vi "Versioned Load BDX.vi"(1 "path":path) -> (8 "Overall":cluster{"Time (s)":dbl, "Distance (ft)":dbl}, 9 "Trajectory Meta":cluster{"Drive Type":T3, "Path Type":T4}, 15 "Current Limit":dbl, 16 "Points out":cluster{"x":dbl, "y":dbl, "th":dbl}[](array[cluster]), 17 "Fields":T7 {"Overrides"."Angle Override" step=5.0; "Overrides"."Velocity Override" step=5.0; "Overrides"."Angular Override" step=5.0; "Angular Limits"."Jerk (deg/s^3)" min=0.0 step=1.0; "Angular Limits"."Accel (deg/s^2)" min=0.0; "Angular Limits"."Velocity (deg/s)" min=0.0}, 20 "Commands out":T8, 21 "Zero V":bool, 24 "Reversals":T11, 25 "Trajectory Data":T1, 26 "Zero Translational Velocity":bool)   [LabVIEW 2025]
uses:
  Types/Full Command Info.ctl
  Types/Single Cmd Info.ctl
  <vilib>/picture/picture.llb/imagedata.ctl
  Types/Overrides.ctl
  Types/Angluar Limits.ctl
  Types/Drive Type.ctl
  Types/Path Type.ctl
  Types/Trajectory Data.ctl
  Types/Segment Type.ctl
  Types/Availible Command systems for auto.ctl
  Types/Limits.ctl
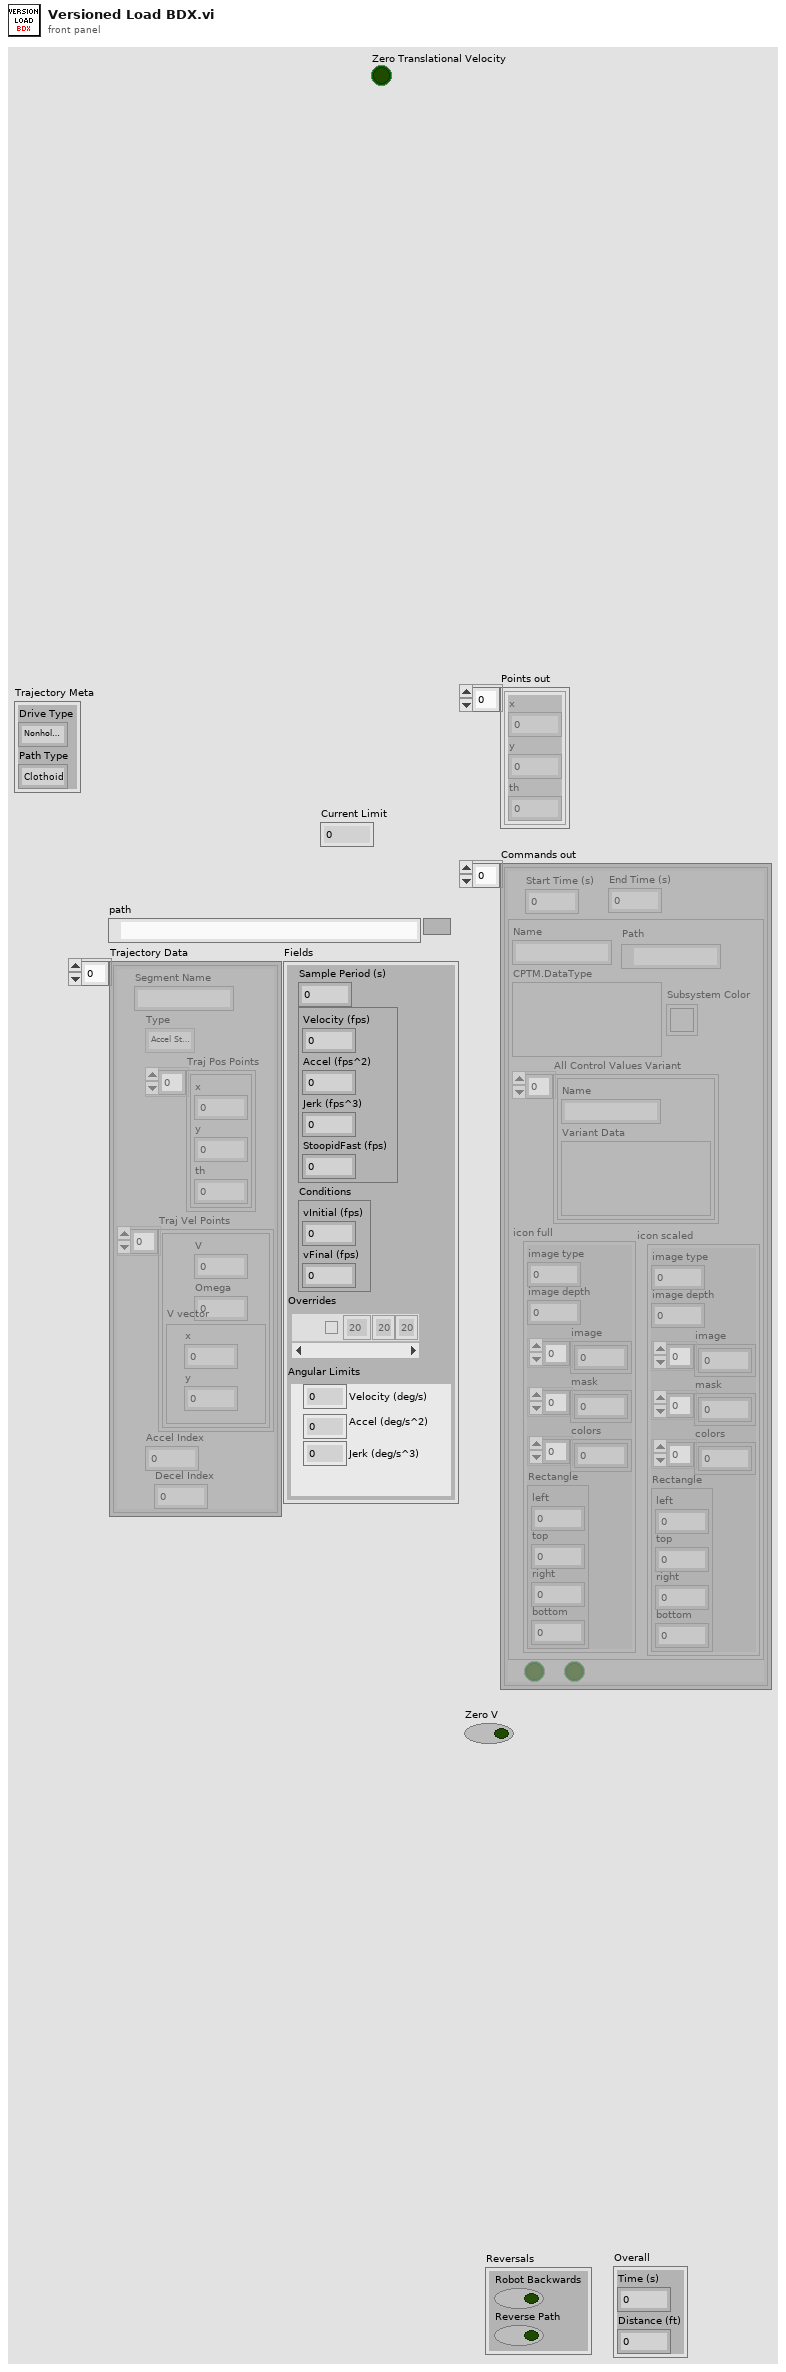
[diagram p1: front panel]
types:
  T1 = typedef "Trajectory Data.ctl" = cluster{"Segment Name":string, "Type":T2, "Traj Pos Points":cluster{"x":dbl, "y":dbl, "th":dbl}[], "Traj Vel Points":cluster{"V":dbl, "Omega":dbl, "V vector":cluster{"y":dbl, "x":dbl}}[], "Accel Index":i32, "Decel Index":i32}[]
  T2 = typedef "Segment Type.ctl" = enum16{"Accel Straight", "Const Straight", "Blend", "Circle", "Bezier"}
  T3 = typedef "Drive Type.ctl" = enum16{"Nonholonomic", "Holonomic"}
  T4 = typedef "Path Type.ctl" = enum16{"Clothoid", "Bezier"}
  T5 = typedef "Overrides.ctl" = cluster{"Count":string, "Angular Override":dbl, "Enabled?":bool, "Velocity Override":dbl, "Angle Override":dbl}[]
  T6 = typedef "Angluar Limits.ctl" = cluster{"Velocity (deg/s)":dbl, "Accel (deg/s^2)":dbl, "Jerk (deg/s^3)":dbl}
  T7 = cluster{"Sample Period (s)":dbl, cluster{"Velocity (fps)":dbl, "Accel (fps^2)":dbl, "Jerk (fps^3)":dbl, "StoopidFast (fps)":dbl}, "Conditions":cluster{"vInitial (fps)":dbl, "vFinal (fps)":dbl}, "Overrides":T5, "Angular Limits":T6}
  T8 = typedef "Full Command Info.ctl" = cluster{"Start Time (s)":dbl, "End Time (s)":dbl, T9, "Visible":bool, "Enabled?":bool}[]
  T9 = typedef "Single Cmd Info.ctl" = cluster{"Name":string, "CPTM.DataType":variant, "All Control Values Variant":cluster{"Name":string, "Variant Data":variant}[], "icon full":T10, "icon scaled":T10, "Path":path, "Subsystem Color":u32}
  T10 = typedef "imagedata.ctl" = cluster{"image type":i32, "image depth":i32, "image":u8[], "mask":u8[], "colors":u32[], "Rectangle":cluster{"left":i16, "top":i16, "right":i16, "bottom":i16}}
  T11 = cluster{"Robot Backwards":bool, "Reverse Path":bool}
  T12 = cluster{"Segment Name":string, "Type":T2, "Traj Pos Points":cluster{"x":dbl, "y":dbl, "th":dbl}[], "Traj Vel Points":cluster{"V":dbl, "Omega":dbl}[], "Accel Index":i32, "Decel Index":i32}[]
  T13 = cluster{"Sample Period (s)":dbl, "Limits 2":cluster{"Velocity (fps)":dbl, "Acceleration (fps^2)":dbl, "Jerk (fps^3)":dbl}, "Conditions":cluster{"vInitial (fps)":dbl, "vFinal (fps)":dbl}, " Acceleration Overrides":cluster{"Angular \nAccelerations":dbl[], "Accel Override Bools":bool[]}}
  T14 = cluster{"Velocity":dbl, "Sample Time":dbl, "Accel":dbl}
  T15 = cluster{"Sample Period (s)":dbl, "Limits":cluster{"Velocity (fps)":dbl, "Acceleration (fps^2)":dbl, "Jerk (fps^3)":dbl}, "Conditions":cluster{"vInitial (fps)":dbl, "vFinal (fps)":dbl}}
  T16 = cluster{"Sample Period (s)":dbl, "Limits":cluster{"Velocity (fps)":dbl, "Acceleration (fps^2)":dbl, "Jerk (fps^3)":dbl}, "Conditions":cluster{"vInitial (fps)":dbl, "vFinal (fps)":dbl}, "Min Rads":dbl[]}
  T17 = typedef "Availible Command systems for auto.ctl" = u16
  T18 = cluster{"Time into Path":dbl, "System":T17, "Item Selected?":bool, "System Selection":T17}[]
  T19 = cluster{"Sample Period (s)":dbl, "Limits 2":cluster{"Velocity (fps)":dbl, "Acceleration (fps^2)":dbl, "Jerk (fps^3)":dbl, "Stoopid Fast":dbl}, "Conditions":cluster{"vInitial (fps)":dbl, "vFinal (fps)":dbl}, " Acceleration Overrides":cluster{"Angular \nAccelerations":dbl[], "Accel Override Bools":bool[]}}
  T20 = cluster{"Sample Period (s)":dbl, "Limits":cluster{"Velocity (fps)":dbl, "Accel (fps^2)":dbl, "Turn Accel (fps^2)":dbl, "Jerk (fps^3)":dbl}, "Conditions":cluster{"vInitial (fps)":dbl, "vFinal (fps)":dbl}, cluster{dbl[], bool[]}}
  T21 = cluster{"Reverse Path":bool, "Robot Backwards":bool}
  T22 = typedef "Limits.ctl" = cluster{"Velocity (fps)":dbl, "Accel (fps^2)":dbl, "Jerk (fps^3)":dbl, "StoopidFast (fps)":dbl}
  T23 = cluster{"Sample Period (s)":dbl, "Limits":T22, "Conditions":cluster{"vInitial (fps)":dbl, "vFinal (fps)":dbl}, "Overrides":T5, "Angular Limits":T6}
  T24 = cluster{"Start Time (s)":dbl, "End Time (s)":dbl, T9, "Visible":bool, "Enabled?":bool}[]
  T25 = cluster{"Velocity":dbl, "Accel":dbl, "Accel":dbl, "Velocity":dbl}
  T26 = cluster{"Velocity (fps)":dbl, "Acceleration (fps^2)":dbl, "Jerk (fps^3)":dbl}
  T27 = cluster{"vInitial (fps)":dbl, "vFinal (fps)":dbl}
  T28 = cluster{"Velocity (fps)":dbl, "Acceleration (fps^2)":dbl, "Jerk (fps^3)":dbl, "Velocity (fps)":dbl}
  T29 = cluster{string, "Angular Multiplier":dbl, bool, "Velocity (fps)":dbl, "Velocity (fps)":dbl}
  T30 = cluster{"Angular \nAccelerations":dbl[], "Accel Override Bools":bool[]}
  T31 = cluster{"Velocity (fps)":dbl, "Acceleration (fps^2)":dbl, "Jerk (fps^3)":dbl, "Stoopid Fast":dbl}
  T32 = cluster{"Velocity (fps)":dbl, "Accel (fps^2)":dbl, "Turn Accel (fps^2)":dbl, "Jerk (fps^3)":dbl}
  T33 = cluster{"Velocity (fps)":dbl, "Accel (fps^2)":dbl, "Jerk (fps^3)":dbl, "StoopidFast (fps)":dbl}
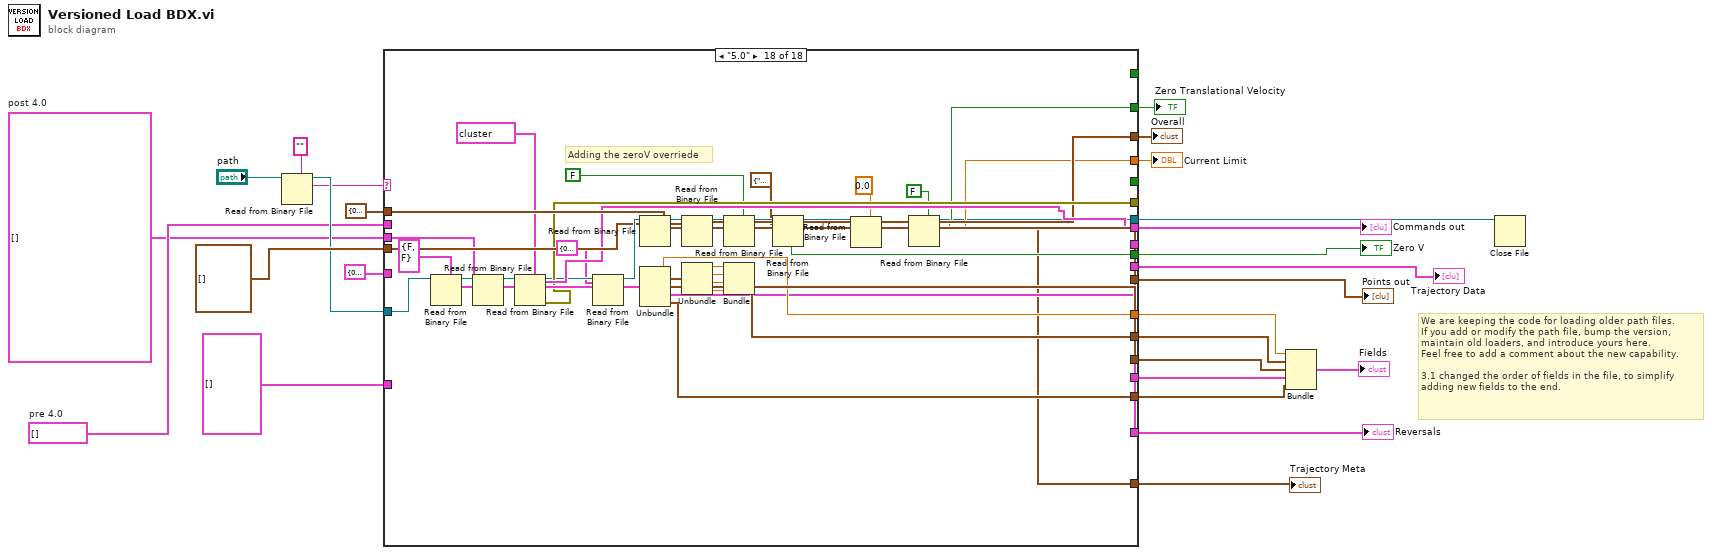
[diagram p0: block diagram]
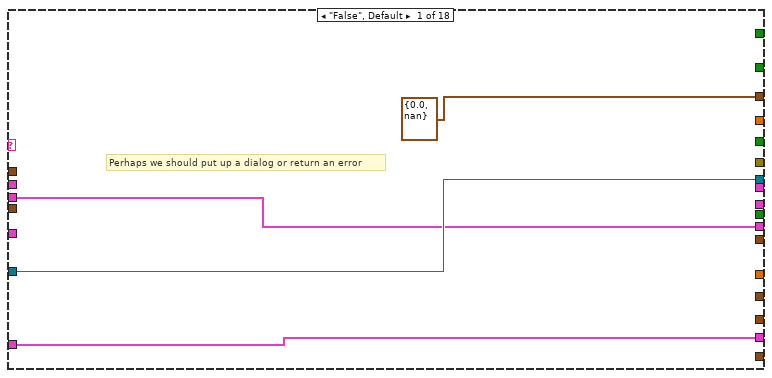
[diagram p2: hidden frame]
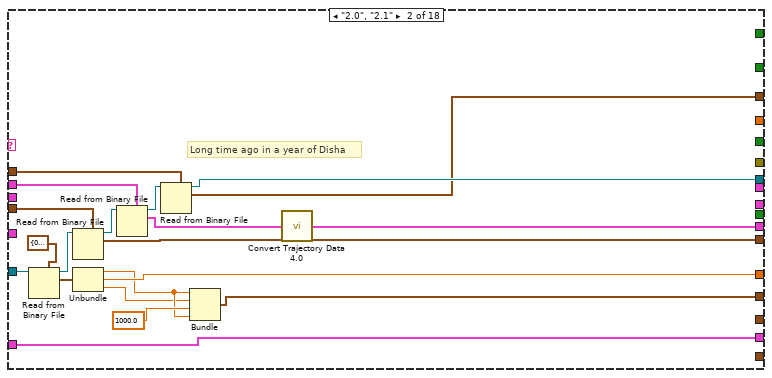
[diagram p3: hidden frame]
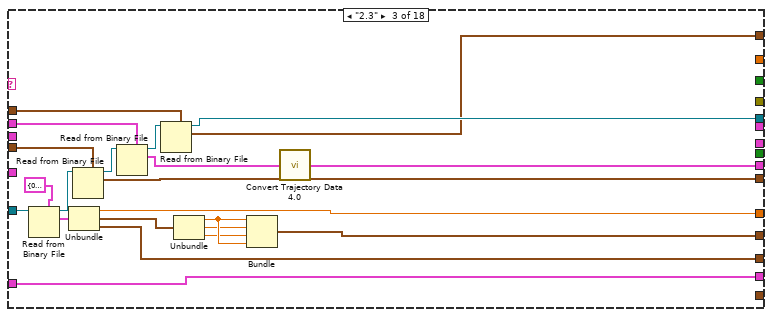
[diagram p4: hidden frame]
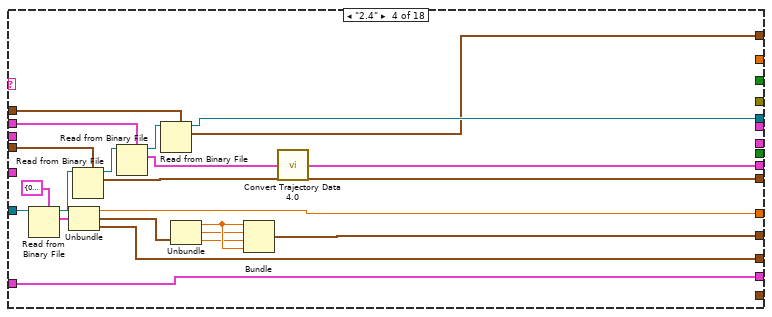
[diagram p5: hidden frame]
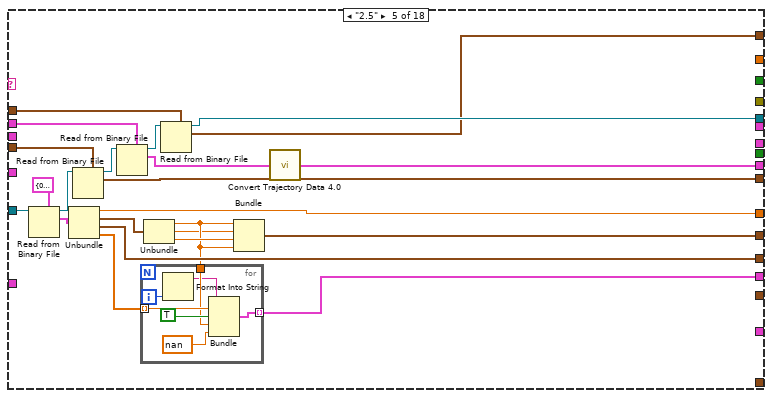
[diagram p6: hidden frame]
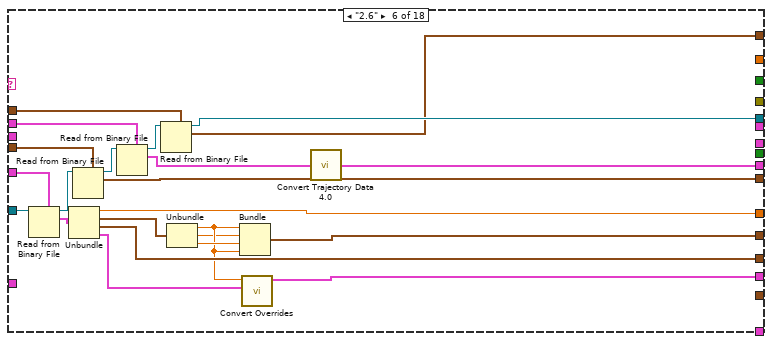
[diagram p7: hidden frame]
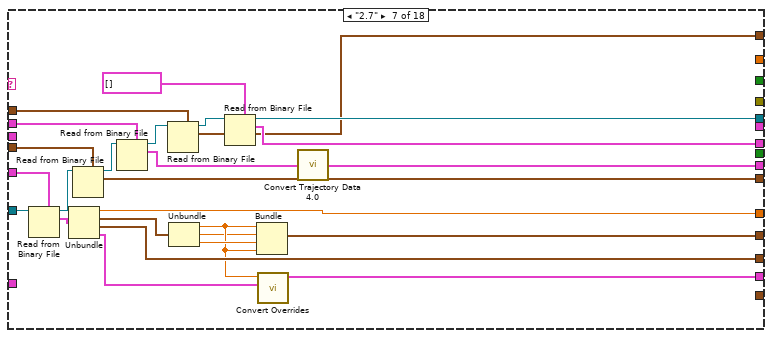
[diagram p8: hidden frame]
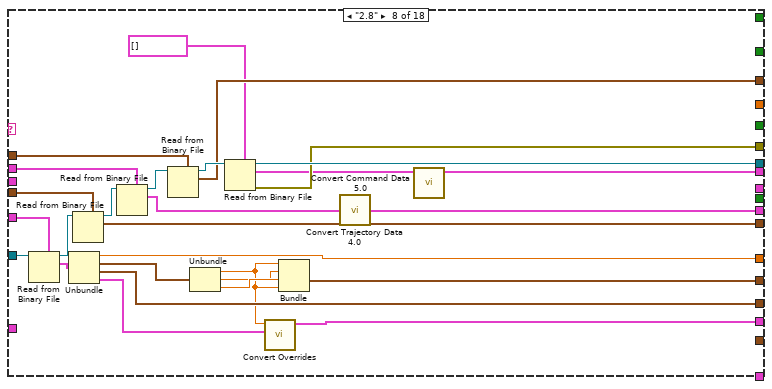
[diagram p9: hidden frame]
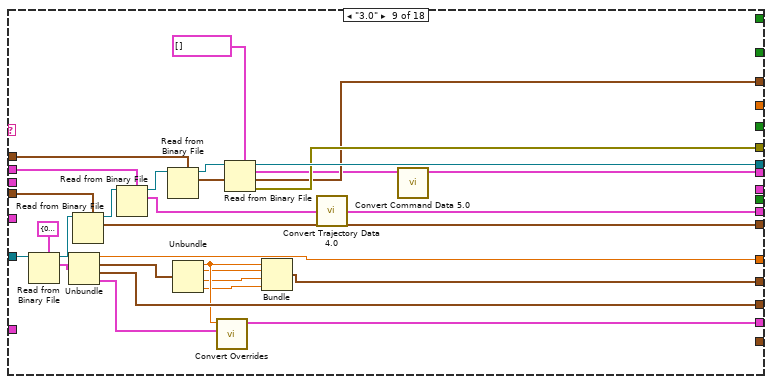
[diagram p10: hidden frame]
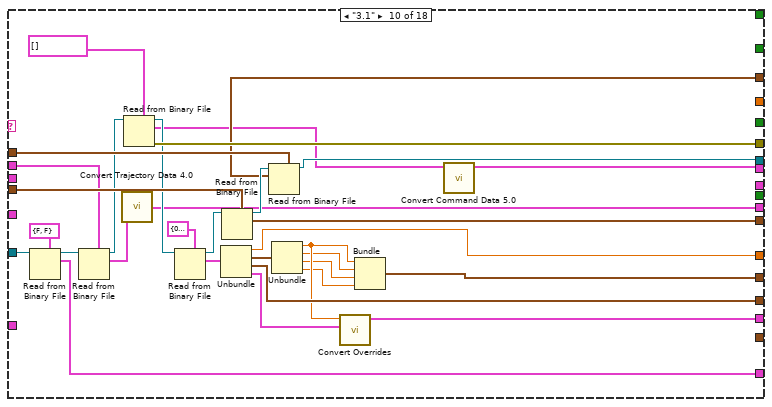
[diagram p11: hidden frame]
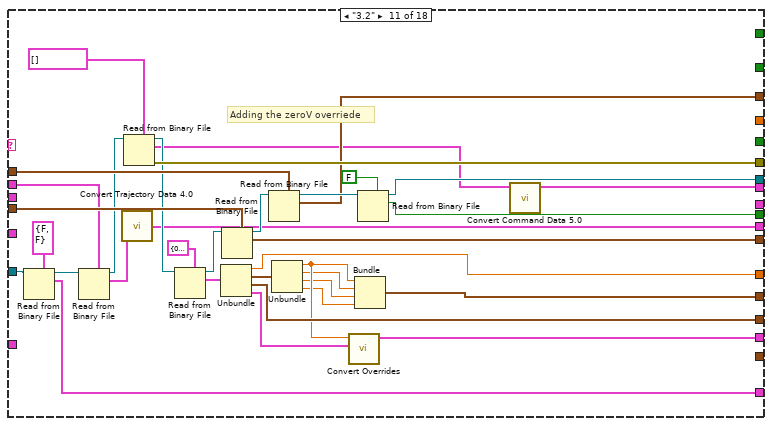
[diagram p12: hidden frame]
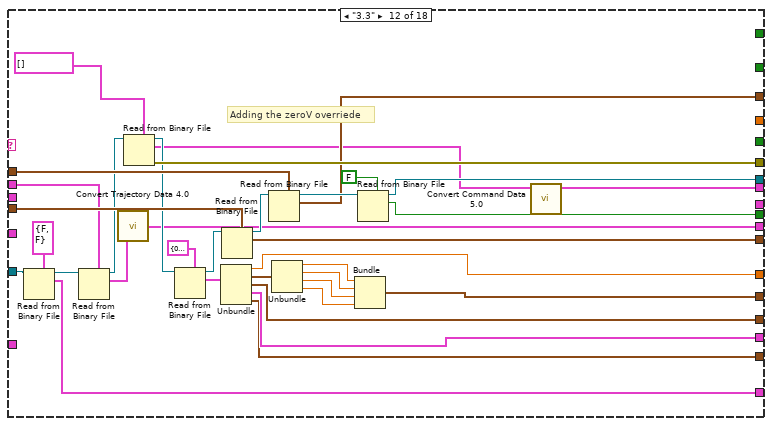
[diagram p13: hidden frame]
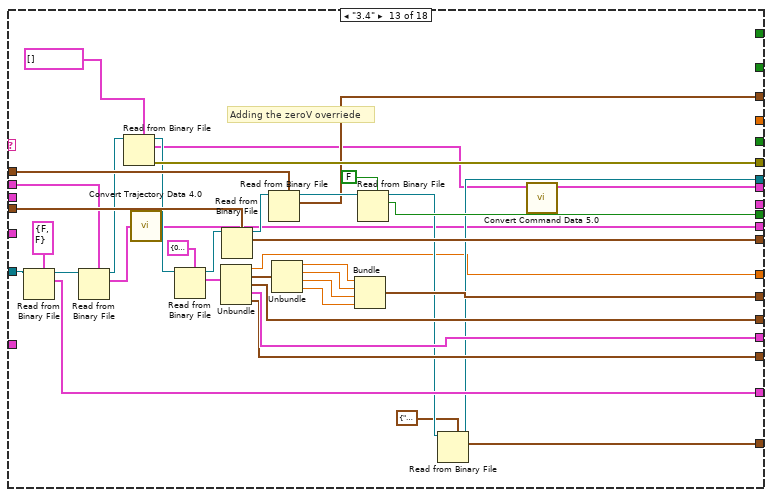
[diagram p14: hidden frame]
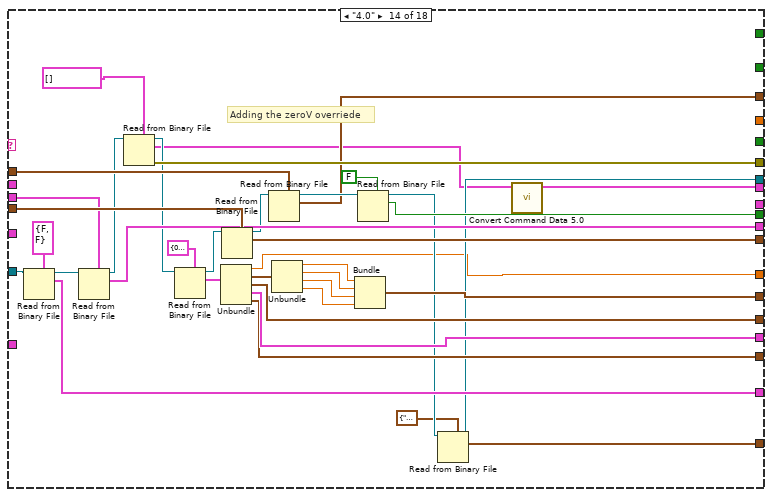
[diagram p15: hidden frame]
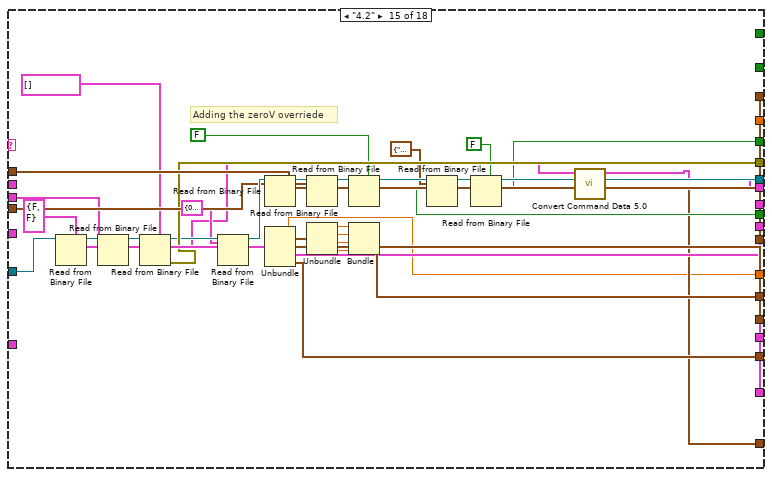
[diagram p16: hidden frame]
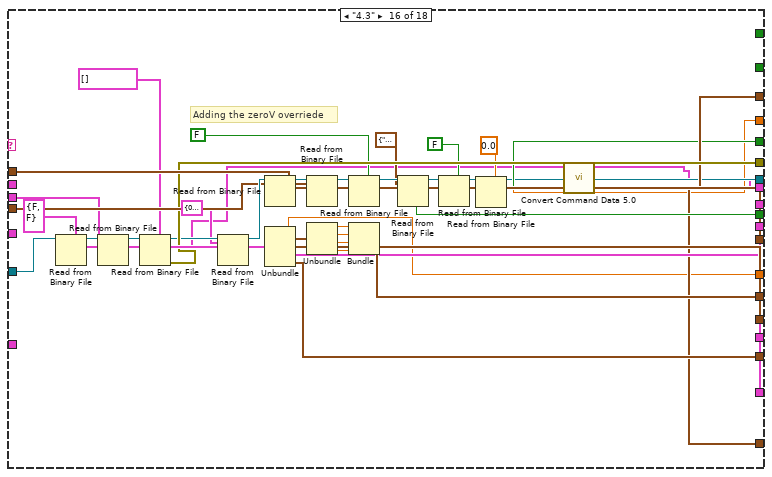
[diagram p17: hidden frame]
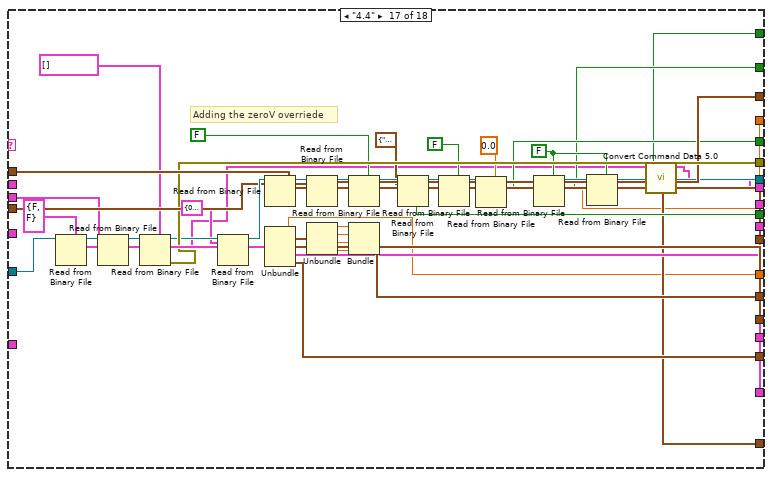
[diagram p18: hidden frame]
diagram:
  w5 = T12 []  # pre 4.0
  w4 = T1 []  # post 4.0
  # "We are keeping the code for loading older path files.\nIf you add or modify the path file, bump the version,\nmaintain old loaders, and introduce yours here.\nFeel free to add a comment about the new capability.\n\n3.1 changed the order of fields in the file, to simplify\nadding new fields to the end."
  n1 = Read from Binary File(5:"" ("String"), 11:"path") -> (2:w11:string, 3:w12:refnum<file>)  [unwired: 4 in, 2 out]
  n2 = case shown="\"5.0\"" w11 {
    tunnel: w12 -> [w30 w49 w71 w93 w116 w146 w172 w200 w229 w253 w288 w323 w361 w399 w439 w482 w530 w571]
    tunnel: cluster{"x":dbl, "y":dbl, "th":dbl}[] [] ("Points in") -> [_ w47 w69 w91 w114 w144 w170 w198 w227 w260 w295 w330 w368 w405 w445 w488 w536 w578]
    tunnel: [_ w46 w68 w90 w113 w143 w169 w197 w226 w259 w294 w329 w367 w404 w444 w487 w535 w577] -> w17
    tunnel: w5 -> [_ w45 w67 w89 w112 w142 w168 w196 w225 w258 w293 w328 w366 _ _ _ _ _]
    tunnel: cluster{"Time (s)":dbl, "Distance (ft)":dbl} {"Time (s)"=0.0, "Distance (ft)"=0.0} ("Cluster 4") -> [_ w43 w65 w87 w110 w140 w166 w194 w223 w257 w292 w327 w365 w403 w443 w486 w534 w576]
    tunnel: [w30 w41 w63 w85 w108 w138 w160 w189 w218 w249 w271 w309 w339 w377 w414 w454 w495 w541] -> w14
    tunnel: [_ w39 w62 w84 w107 w137 w164 w174 w202 w233 w263 w298 w333 w372 w408 w448 w491 w558] -> w23
    tunnel: [_ w35 w56 w77 w101 w132 w154 w186 w208 w241 w277 w315 w353 w391 w431 w474 w522 w563] -> w24
    tunnel: [_ _ w61 w83 w106 w136 w163 w192 w221 w256 w291 w326 w364 w402 w442 w485 w533 w575] -> w25
    tunnel: [w29 w34 w55 w76 w100 w130 w151 w183 w214 w245 w281 w304 w343 w381 w421 w464 w512 w552] -> w26
    tunnel: [w27 w31 w51 w73 w95 w125 w148 w178 w206 w235 w267 w302 w337 w401 w441 w484 w532 w574] -> w3
    tunnel: [_ _ _ _ _ _ w159 _ _ _ _ _ _ _ _ _ _ _] -> _
    tunnel: [_ _ _ _ _ _ _ w175 w203 w231 w264 w299 w334 w371 w409 w449 w493 w573] -> w18
    tunnel: [_ _ _ _ _ _ _ w188 w217 w254 w289 w324 w362 w400 w440 w483 w531 w572] -> _
    tunnel: T13 {"Sample Period (s)"=0.0, "Limits 2"={"Velocity (fps)"=0.0, "Acceleration (fps^2)"=0.0, "Jerk (fps^3)"=0.0}, "Conditions"={"vInitial (fps)"=0.0, "vFinal (fps)"=0.0}, " Acceleration Overrides"={"Angular \nAccelerations"=[], "Accel Override Bools"=[]}} ("Cluster") -> [_ _ _ _ _ w134 w157 w184 _ _ _ _ _ _ _ _ _ _]
    tunnel: [_ _ _ _ _ _ _ _ _ w244 w280 w317 w355 w393 w433 w476 w524 w565] -> w20
    tunnel: T5 [] ("Overrides") -> [w29 w34 w55 w76 _ _ _ _ _ _ _ _ _ _ _ _ _ _]
    tunnel: [_ _ _ _ _ _ _ _ _ _ w269 w307 w346 w384 w424 w467 w515 w555] -> w21
    tunnel: [cluster{"Time (s)":dbl, "Distance (ft)":dbl} {"Time (s)"=0.0, "Distance (ft)"=nan} ("Cluster 4") w32 w52 w74 w96 w126 w149 w179 w207 w236 w268 w306 w345 w383 w423 w466 w514 w554] -> w9
    tunnel: [_ _ _ _ _ _ _ _ _ _ _ w303 w342 w380 w420 w463 w511 w551] -> w7
    tunnel: [_ _ _ _ _ _ _ _ _ _ _ _ w338 w376 w417 w460 w508 w548] -> w6
    tunnel: w4 -> [w27 _ _ _ _ _ _ _ _ _ _ _ _ w375 w416 w459 w507 w547]
    tunnel: [_ _ _ _ _ _ _ _ _ _ _ _ _ _ w412 w456 w504 _] -> _
    tunnel: [_ _ _ _ _ _ _ _ _ _ _ _ _ _ _ w452 w501 w545] -> w2
    tunnel: [_ _ _ _ _ _ _ _ _ _ _ _ _ _ _ _ w497 w542] -> w1
    tunnel: [_ _ _ _ _ _ _ _ _ _ _ _ _ _ _ _ w496 _] -> _
    frame "False", Default {
      # "Perhaps we should put up a dialog or return an error"
    }
    frame "2.0", "2.1" {
      # "Long time ago in a year of Disha"
      n3 = Read from Binary File(5:T14 {"Velocity"=0.0, "Sample Time"=0.0, "Accel"=0.0}, 11:w49) -> (2:w50:T14, 3:w48:refnum<file>)  [unwired: 4 in, 2 out]
      n4 = Read from Binary File(5:w47, 11:w48) -> (2:w46:cluster{"x":dbl, "y":dbl, "th":dbl}[], 3:w44:refnum<file>)  [unwired: 4 in, 2 out]
      n5 = Unbundle(w50) -> ("Velocity"=w36:dbl, "Sample Time"=w39:dbl, "Accel"=w33:dbl)
      n6 = Read from Binary File(5:w45, 11:w44) -> (2:w37:T12, 3:w42:refnum<file>)  [unwired: 4 in, 2 out]
      n7 = Read from Binary File(5:w43, 11:w42) -> (2:w32:cluster{"Time (s)":dbl, "Distance (ft)":dbl}, 3:w41:refnum<file>)  [unwired: 4 in, 2 out]
      n8 = Bundle("Velocity"=w36, "Accel"=w33, "Accel"=1000.0, "Velocity"=w36) -> (w35:T25)  [unwired: 1 in]
      n9 = call "Convert Trajectory Data 4.0.vi"("pre 4.0"=w37) -> ("post 4.0"=w31:T1)
    }
    frame "2.3" {
      n10 = Read from Binary File(5:T15 {"Sample Period (s)"=0.0, "Limits"={"Velocity (fps)"=0.0, "Acceleration (fps^2)"=0.0, "Jerk (fps^3)"=0.0}, "Conditions"={"vInitial (fps)"=0.0, "vFinal (fps)"=0.0}}, 11:w71) -> (2:w72:T15, 3:w70:refnum<file>)  [unwired: 4 in, 2 out]
      n11 = Unbundle(w72) -> ("Sample Period (s)"=w62:dbl, "Limits"=w53:T26, "Conditions"=w61:T27)
      n12 = Read from Binary File(5:w69, 11:w70) -> (2:w68:cluster{"x":dbl, "y":dbl, "th":dbl}[], 3:w66:refnum<file>)  [unwired: 4 in, 2 out]
      n13 = Read from Binary File(5:w67, 11:w66) -> (2:w59:T12, 3:w64:refnum<file>)  [unwired: 4 in, 2 out]
      n14 = Read from Binary File(5:w65, 11:w64) -> (2:w52:cluster{"Time (s)":dbl, "Distance (ft)":dbl}, 3:w63:refnum<file>)  [unwired: 4 in, 2 out]
      n15 = Unbundle(w53) -> ("Velocity (fps)"=w58:dbl, "Acceleration (fps^2)"=w54:dbl, "Jerk (fps^3)"=w57:dbl)
      n16 = Bundle("Velocity (fps)"=w58, "Acceleration (fps^2)"=w54, "Jerk (fps^3)"=w57, "Velocity (fps)"=w58) -> (w56:T28)  [unwired: 1 in]
      n17 = call "Convert Trajectory Data 4.0.vi"("pre 4.0"=w59) -> ("post 4.0"=w51:T1)
    }
    frame "2.4" {
      n18 = Read from Binary File(5:T15 {"Sample Period (s)"=0.0, "Limits"={"Velocity (fps)"=0.0, "Acceleration (fps^2)"=0.0, "Jerk (fps^3)"=0.0}, "Conditions"={"vInitial (fps)"=0.0, "vFinal (fps)"=0.0}}, 11:w93) -> (2:w94:T15, 3:w92:refnum<file>)  [unwired: 4 in, 2 out]
      n19 = Unbundle(w94) -> ("Sample Period (s)"=w84:dbl, "Limits"=w78:T26, "Conditions"=w83:T27)
      n20 = Read from Binary File(5:w91, 11:w92) -> (2:w90:cluster{"x":dbl, "y":dbl, "th":dbl}[], 3:w88:refnum<file>)  [unwired: 4 in, 2 out]
      n21 = Read from Binary File(5:w89, 11:w88) -> (2:w81:T12, 3:w86:refnum<file>)  [unwired: 4 in, 2 out]
      n22 = Read from Binary File(5:w87, 11:w86) -> (2:w74:cluster{"Time (s)":dbl, "Distance (ft)":dbl}, 3:w85:refnum<file>)  [unwired: 4 in, 2 out]
      n23 = Unbundle(w78) -> ("Velocity (fps)"=w80:dbl, "Acceleration (fps^2)"=w75:dbl, "Jerk (fps^3)"=w79:dbl)
      n24 = Bundle("Velocity (fps)"=w80, "Acceleration (fps^2)"=w75, "Jerk (fps^3)"=w79, "Velocity (fps)"=w80) -> (w77:T28)  [unwired: 1 in]
      n25 = call "Convert Trajectory Data 4.0.vi"("pre 4.0"=w81) -> ("post 4.0"=w73:T1)
    }
    frame "2.5" {
      n26 = Read from Binary File(5:T16 {"Sample Period (s)"=0.0, "Limits"={"Velocity (fps)"=0.0, "Acceleration (fps^2)"=0.0, "Jerk (fps^3)"=0.0}, "Conditions"={"vInitial (fps)"=0.0, "vFinal (fps)"=0.0}, "Min Rads"=[20.0, 20.0, 20.0, 20.0, 20.0]}, 11:w116) -> (2:w117:T16, 3:w115:refnum<file>)  [unwired: 4 in, 2 out]
      n27 = Unbundle(w117) -> ("Sample Period (s)"=w107:dbl, "Limits"=w102:T26, "Conditions"=w106:T27, "Min Rads"=w99:dbl[])
      n28 = Read from Binary File(5:w114, 11:w115) -> (2:w113:cluster{"x":dbl, "y":dbl, "th":dbl}[], 3:w111:refnum<file>)  [unwired: 4 in, 2 out]
      n29 = Read from Binary File(5:w112, 11:w111) -> (2:w104:T12, 3:w109:refnum<file>)  [unwired: 4 in, 2 out]
      n30 = Unbundle(w102) -> ("Velocity (fps)"=w98:dbl, "Acceleration (fps^2)"=w97:dbl, "Jerk (fps^3)"=w103:dbl)
      n31 = for {
        tunnel: [w123] -> w100 mode=indexing
        tunnel: w99 -> [w122] mode=indexing
        tunnel: w98 -> [w121]
        i -> [w120]
        n32 = Format Into String(w120) -> (resulting string=w119:string)  [unwired: 3 in, 1 out]
        n33 = Bundle(w119, "Angular Multiplier"=w122, TRUE, "Velocity (fps)"=w121, "Velocity (fps)"=nan) -> (w123:T29)  [unwired: 1 in]
      }
      n34 = Read from Binary File(5:w110, 11:w109) -> (2:w96:cluster{"Time (s)":dbl, "Distance (ft)":dbl}, 3:w108:refnum<file>)  [unwired: 4 in, 2 out]
      n35 = Bundle("Velocity (fps)"=w98, "Acceleration (fps^2)"=w97, "Jerk (fps^3)"=w103, "Velocity (fps)"=w98) -> (w101:T28)  [unwired: 1 in]
      n36 = call "Convert Trajectory Data 4.0.vi"("pre 4.0"=w104) -> ("post 4.0"=w95:T1)
    }
    frame "2.6" {
      n37 = Read from Binary File(5:w134, 11:w146) -> (2:w147:T13, 3:w145:refnum<file>)  [unwired: 4 in, 2 out]
      n38 = Unbundle(w147) -> ("Sample Period (s)"=w137:dbl, "Limits 2"=w131:T26, "Conditions"=w136:T27, "Acceleration Overrides"=w128:T30)
      n39 = Read from Binary File(5:w144, 11:w145) -> (2:w143:cluster{"x":dbl, "y":dbl, "th":dbl}[], 3:w141:refnum<file>)  [unwired: 4 in, 2 out]
      n40 = Read from Binary File(5:w142, 11:w141) -> (2:w135:T12, 3:w139:refnum<file>)  [unwired: 4 in, 2 out]
      n41 = Read from Binary File(5:w140, 11:w139) -> (2:w126:cluster{"Time (s)":dbl, "Distance (ft)":dbl}, 3:w138:refnum<file>)  [unwired: 4 in, 2 out]
      n42 = Unbundle(w131) -> ("Velocity (fps)"=w129:dbl, "Acceleration (fps^2)"=w127:dbl, "Jerk (fps^3)"=w133:dbl)
      n43 = Bundle("Velocity (fps)"=w129, "Acceleration (fps^2)"=w127, "Jerk (fps^3)"=w133, "Velocity (fps)"=w129) -> (w132:T28)  [unwired: 1 in]
      n44 = call "Convert Overrides.vi"("Cluster"=w128, "Velocity (fps)"=w129) -> ("Overrides"=w130:T5)  [unwired: 9 in]
      n45 = call "Convert Trajectory Data 4.0.vi"("pre 4.0"=w135) -> ("post 4.0"=w125:T1)
    }
    frame "2.7" {
      n46 = Read from Binary File(5:w157, 11:w172) -> (2:w173:T13, 3:w171:refnum<file>)  [unwired: 4 in, 2 out]
      n47 = Unbundle(w173) -> ("Sample Period (s)"=w164:dbl, "Limits 2"=w155:T26, "Conditions"=w163:T27, "Acceleration Overrides"=w152:T30)
      n48 = Read from Binary File(5:w170, 11:w171) -> (2:w169:cluster{"x":dbl, "y":dbl, "th":dbl}[], 3:w167:refnum<file>)  [unwired: 4 in, 2 out]
      n49 = Read from Binary File(5:w168, 11:w167) -> (2:w162:T12, 3:w165:refnum<file>)  [unwired: 4 in, 2 out]
      n50 = Read from Binary File(5:w166, 11:w165) -> (2:w149:cluster{"Time (s)":dbl, "Distance (ft)":dbl}, 3:w161:refnum<file>)  [unwired: 4 in, 2 out]
      n51 = Unbundle(w155) -> ("Velocity (fps)"=w153:dbl, "Acceleration (fps^2)"=w150:dbl, "Jerk (fps^3)"=w156:dbl)
      n52 = Read from Binary File(5:T18 [] ("Commands"), 11:w161) -> (2:w159:T18, 3:w160:refnum<file>)  [unwired: 4 in, 2 out]
      n53 = Bundle("Velocity (fps)"=w153, "Acceleration (fps^2)"=w150, "Jerk (fps^3)"=w156, "Velocity (fps)"=w153) -> (w154:T28)  [unwired: 1 in]
      n54 = call "Convert Overrides.vi"("Cluster"=w152, "Velocity (fps)"=w153) -> ("Overrides"=w151:T5)  [unwired: 9 in]
      n55 = call "Convert Trajectory Data 4.0.vi"("pre 4.0"=w162) -> ("post 4.0"=w148:T1)
    }
    frame "2.8" {
      n56 = Read from Binary File(5:w184, 11:w200) -> (2:w201:T13, 3:w199:refnum<file>)  [unwired: 4 in, 2 out]
      n57 = Unbundle(w201) -> ("Sample Period (s)"=w174:dbl, "Limits 2"=w187:T26, "Conditions"=w192:T27, "Acceleration Overrides"=w181:T30)
      n58 = Read from Binary File(5:w198, 11:w199) -> (2:w197:cluster{"x":dbl, "y":dbl, "th":dbl}[], 3:w195:refnum<file>)  [unwired: 4 in, 2 out]
      n59 = Read from Binary File(5:w196, 11:w195) -> (2:w191:T12, 3:w193:refnum<file>)  [unwired: 4 in, 2 out]
      n60 = Read from Binary File(5:w194, 11:w193) -> (2:w179:cluster{"Time (s)":dbl, "Distance (ft)":dbl}, 3:w190:refnum<file>)  [unwired: 4 in, 2 out]
      n61 = Unbundle(w187) -> ("Velocity (fps)"=w182:dbl, "Acceleration (fps^2)"=w180:dbl, "Jerk (fps^3)"=w185:dbl)
      n62 = Read from Binary File(5:cluster{"Time (s)":dbl, T9, bool}[] [] ("Commands in"), 11:w190) -> (0:w188:errorcluster, 2:w176:cluster{"Time (s)":dbl, T9, bool}[], 3:w189:refnum<file>)  [unwired: 4 in, 1 out]
      n63 = call "Convert Overrides.vi"("Cluster"=w181, "Velocity (fps)"=w182) -> ("Overrides"=w183:T5)  [unwired: 9 in]
      n64 = Bundle("Velocity (fps)"=w182, "Acceleration (fps^2)"=w180, "Jerk (fps^3)"=w185, "Velocity (fps)"=w182) -> (w186:T28)  [unwired: 1 in]
      n65 = call "Convert Trajectory Data 4.0.vi"("pre 4.0"=w191) -> ("post 4.0"=w178:T1)
      n66 = call "Convert Command Data 5.0.vi"("Pre 5.0 Command Data"=w176) -> ("5.0 Command Data"=w175:T8)  [unwired: 10 in]
    }
    frame "3.0" {
      n67 = Read from Binary File(5:T19 {"Sample Period (s)"=0.0, "Limits 2"={"Velocity (fps)"=0.0, "Acceleration (fps^2)"=0.0, "Jerk (fps^3)"=0.0, "Stoopid Fast"=0.0}, "Conditions"={"vInitial (fps)"=0.0, "vFinal (fps)"=0.0}, " Acceleration Overrides"={"Angular \nAccelerations"=[], "Accel Override Bools"=[]}} ("Cluster"), 11:w229) -> (2:w230:T19, 3:w228:refnum<file>)  [unwired: 4 in, 2 out]
      n68 = Unbundle(w230) -> ("Sample Period (s)"=w202:dbl, "Limits 2"=w209:T31, "Conditions"=w221:T27, "Acceleration Overrides"=w215:T30)
      n69 = Read from Binary File(5:w227, 11:w228) -> (2:w226:cluster{"x":dbl, "y":dbl, "th":dbl}[], 3:w224:refnum<file>)  [unwired: 4 in, 2 out]
      n70 = Read from Binary File(5:w225, 11:w224) -> (2:w220:T12, 3:w222:refnum<file>)  [unwired: 4 in, 2 out]
      n71 = Read from Binary File(5:w223, 11:w222) -> (2:w207:cluster{"Time (s)":dbl, "Distance (ft)":dbl}, 3:w219:refnum<file>)  [unwired: 4 in, 2 out]
      n72 = Unbundle(w209) -> ("Velocity (fps)"=w213:dbl, "Acceleration (fps^2)"=w212:dbl, "Jerk (fps^3)"=w211:dbl, "Stoopid Fast"=w210:dbl)
      n73 = call "Convert Overrides.vi"("Cluster"=w215, "Velocity (fps)"=w213) -> ("Overrides"=w214:T5)  [unwired: 9 in]
      n74 = Read from Binary File(5:cluster{"Time (s)":dbl, T9, bool}[] [] ("Commands in"), 11:w219) -> (0:w217:errorcluster, 2:w204:cluster{"Time (s)":dbl, T9, bool}[], 3:w218:refnum<file>)  [unwired: 4 in, 1 out]
      n75 = Bundle("Velocity (fps)"=w213, "Acceleration (fps^2)"=w212, "Jerk (fps^3)"=w211, "Stoopid Fast"=w210) -> (w208:T31)  [unwired: 1 in]
      n76 = call "Convert Trajectory Data 4.0.vi"("pre 4.0"=w220) -> ("post 4.0"=w206:T1)
      n77 = call "Convert Command Data 5.0.vi"("Pre 5.0 Command Data"=w204) -> ("5.0 Command Data"=w203:T8)  [unwired: 10 in]
    }
    frame "3.1" {
      n78 = Read from Binary File(5:T21 {"Reverse Path"=FALSE, "Robot Backwards"=FALSE} ("Cluster"), 11:w253) -> (2:w244:T21, 3:w250:refnum<file>)  [unwired: 4 in, 2 out]
      n79 = Read from Binary File(5:w258, 11:w250) -> (2:w255:T12, 3:w248:refnum<file>)  [unwired: 4 in, 2 out]
      n80 = call "Convert Trajectory Data 4.0.vi"("pre 4.0"=w255) -> ("post 4.0"=w235:T1)
      n81 = Read from Binary File(5:cluster{"Time (s)":dbl, T9, bool}[] [] ("Commands in"), 11:w248) -> (0:w254:errorcluster, 2:w232:cluster{"Time (s)":dbl, T9, bool}[], 3:w247:refnum<file>)  [unwired: 4 in, 1 out]
      n82 = Read from Binary File(5:T20 {"Sample Period (s)"=0.0, "Limits"={"Velocity (fps)"=0.0, "Accel (fps^2)"=0.0, "Turn Accel (fps^2)"=15.0, "Jerk (fps^3)"=0.0}, "Conditions"={"vInitial (fps)"=0.0, "vFinal (fps)"=0.0}, {[], []}} ("Cluster 2"), 11:w247) -> (2:w262:T20, 3:w261:refnum<file>)  [unwired: 4 in, 2 out]
      n83 = Unbundle(w262) -> ("Sample Period (s)"=w233:dbl, "Limits"=w243:T32, "Conditions"=w256:T27, w246:cluster{dbl[], bool[]})
      n84 = Read from Binary File(5:w260, 11:w261) -> (2:w259:cluster{"x":dbl, "y":dbl, "th":dbl}[], 3:w251:refnum<file>)  [unwired: 4 in, 2 out]
      n85 = Read from Binary File(5:w257, 11:w251) -> (2:w236:cluster{"Time (s)":dbl, "Distance (ft)":dbl}, 3:w249:refnum<file>)  [unwired: 4 in, 2 out]
      n86 = Unbundle(w243) -> ("Velocity (fps)"=w240:dbl, "Accel (fps^2)"=w239:dbl, "Turn Accel (fps^2)"=w238:dbl, "Jerk (fps^3)"=w237:dbl)
      n87 = call "Convert Overrides.vi"("Cluster"=w246, "Velocity (fps)"=w240) -> ("Overrides"=w245:T5)  [unwired: 9 in]
      n88 = Bundle("Velocity (fps)"=w240, "Accel (fps^2)"=w239, "Turn Accel (fps^2)"=w238, "Jerk (fps^3)"=w237) -> (w241:T32)  [unwired: 1 in]
      n89 = call "Convert Command Data 5.0.vi"("Pre 5.0 Command Data"=w232) -> ("5.0 Command Data"=w231:T8)  [unwired: 10 in]
    }
    frame "3.2" {
      # "Adding the zeroV overriede"
      n90 = Read from Binary File(5:T11 {"Robot Backwards"=FALSE, "Reverse Path"=FALSE} ("Cluster"), 11:w288) -> (2:w280:T11, 3:w285:refnum<file>)  [unwired: 4 in, 2 out]
      n91 = Read from Binary File(5:w293, 11:w285) -> (2:w290:T12, 3:w284:refnum<file>)  [unwired: 4 in, 2 out]
      n92 = call "Convert Trajectory Data 4.0.vi"("pre 4.0"=w290) -> ("post 4.0"=w267:T1)
      n93 = Read from Binary File(5:cluster{"Time (s)":dbl, T9, bool}[] [] ("Commands in"), 11:w284) -> (0:w289:errorcluster, 2:w265:cluster{"Time (s)":dbl, T9, bool}[], 3:w283:refnum<file>)  [unwired: 4 in, 1 out]
      n94 = Read from Binary File(5:T20 {"Sample Period (s)"=0.0, "Limits"={"Velocity (fps)"=0.0, "Accel (fps^2)"=0.0, "Turn Accel (fps^2)"=15.0, "Jerk (fps^3)"=0.0}, "Conditions"={"vInitial (fps)"=0.0, "vFinal (fps)"=0.0}, {[], []}} ("Cluster 2"), 11:w283) -> (2:w297:T20, 3:w296:refnum<file>)  [unwired: 4 in, 2 out]
      n95 = Unbundle(w297) -> ("Sample Period (s)"=w263:dbl, "Limits"=w279:T32, "Conditions"=w291:T27, w282:cluster{dbl[], bool[]})
      n96 = Read from Binary File(5:w295, 11:w296) -> (2:w294:cluster{"x":dbl, "y":dbl, "th":dbl}[], 3:w286:refnum<file>)  [unwired: 4 in, 2 out]
      n97 = Read from Binary File(5:w292, 11:w286) -> (2:w268:cluster{"Time (s)":dbl, "Distance (ft)":dbl}, 3:w272:refnum<file>)  [unwired: 4 in, 2 out]
      n98 = Unbundle(w279) -> ("Velocity (fps)"=w276:dbl, "Accel (fps^2)"=w275:dbl, "Turn Accel (fps^2)"=w274:dbl, "Jerk (fps^3)"=w273:dbl)
      n99 = call "Convert Overrides.vi"("Cluster"=w282, "Velocity (fps)"=w276) -> ("Overrides"=w281:T5)  [unwired: 9 in]
      n100 = Bundle("Velocity (fps)"=w276, "Accel (fps^2)"=w275, "Turn Accel (fps^2)"=w274, "Jerk (fps^3)"=w273) -> (w277:T32)  [unwired: 1 in]
      n101 = Read from Binary File(5:FALSE, 11:w272) -> (2:w269:bool, 3:w271:refnum<file>)  [unwired: 4 in, 2 out]
      n102 = call "Convert Command Data 5.0.vi"("Pre 5.0 Command Data"=w265) -> ("5.0 Command Data"=w264:T8)  [unwired: 10 in]
    }
    frame "3.3" {
      # "Adding the zeroV overriede"
      n103 = Read from Binary File(5:T11 {"Robot Backwards"=FALSE, "Reverse Path"=FALSE} ("Cluster"), 11:w323) -> (2:w317:T11, 3:w320:refnum<file>)  [unwired: 4 in, 2 out]
      n104 = Read from Binary File(5:w328, 11:w320) -> (2:w325:T12, 3:w319:refnum<file>)  [unwired: 4 in, 2 out]
      n105 = call "Convert Trajectory Data 4.0.vi"("pre 4.0"=w325) -> ("post 4.0"=w302:T1)
      n106 = Read from Binary File(5:cluster{"Time (s)":dbl, T9, bool}[] [] ("Commands in"), 11:w319) -> (0:w324:errorcluster, 2:w300:cluster{"Time (s)":dbl, T9, bool}[], 3:w318:refnum<file>)  [unwired: 4 in, 1 out]
      n107 = Read from Binary File(5:T23 {"Sample Period (s)"=0.0, "Limits"={"Velocity (fps)"=0.0, "Accel (fps^2)"=0.0, "Jerk (fps^3)"=0.0, "StoopidFast (fps)"=0.0}, "Conditions"={"vInitial (fps)"=0.0, "vFinal (fps)"=0.0}, "Overrides"=[], "Angular Limits"={"Velocity (deg/s)"=0.0, "Accel (deg/s^2)"=0.0, "Jerk (deg/s^3)"=0.0}} ("output cluster"), 11:w318) -> (2:w332:T23, 3:w331:refnum<file>)  [unwired: 4 in, 2 out]
      n108 = Unbundle(w332) -> ("Sample Period (s)"=w298:dbl, "Limits"=w316:T22, "Conditions"=w326:T27, "Overrides"=w304:T5, "Angular Limits"=w303:T6)
      n109 = Read from Binary File(5:w330, 11:w331) -> (2:w329:cluster{"x":dbl, "y":dbl, "th":dbl}[], 3:w321:refnum<file>)  [unwired: 4 in, 2 out]
      n110 = Read from Binary File(5:w327, 11:w321) -> (2:w306:cluster{"Time (s)":dbl, "Distance (ft)":dbl}, 3:w310:refnum<file>)  [unwired: 4 in, 2 out]
      n111 = Unbundle(w316) -> ("Velocity (fps)"=w314:dbl, "Accel (fps^2)"=w313:dbl, "Jerk (fps^3)"=w312:dbl, "StoopidFast (fps)"=w311:dbl)
      n112 = Bundle("Velocity (fps)"=w314, "Accel (fps^2)"=w313, "Jerk (fps^3)"=w312, "StoopidFast (fps)"=w311) -> (w315:T33)  [unwired: 1 in]
      n113 = Read from Binary File(5:FALSE, 11:w310) -> (2:w307:bool, 3:w309:refnum<file>)  [unwired: 4 in, 2 out]
      n114 = call "Convert Command Data 5.0.vi"("Pre 5.0 Command Data"=w300) -> ("5.0 Command Data"=w299:T8)  [unwired: 10 in]
    }
    frame "3.4" {
      # "Adding the zeroV overriede"
      n115 = Read from Binary File(5:T11 {"Robot Backwards"=FALSE, "Reverse Path"=FALSE} ("Cluster"), 11:w361) -> (2:w355:T11, 3:w358:refnum<file>)  [unwired: 4 in, 2 out]
      n116 = Read from Binary File(5:w366, 11:w358) -> (2:w363:T12, 3:w357:refnum<file>)  [unwired: 4 in, 2 out]
      n117 = Read from Binary File(5:cluster{"Time (s)":dbl, T9, bool}[] [] ("Commands in"), 11:w357) -> (0:w362:errorcluster, 2:w335:cluster{"Time (s)":dbl, T9, bool}[], 3:w356:refnum<file>)  [unwired: 4 in, 1 out]
      n118 = call "Convert Trajectory Data 4.0.vi"("pre 4.0"=w363) -> ("post 4.0"=w337:T1)
      n119 = Read from Binary File(5:T23 {"Sample Period (s)"=0.0, "Limits"={"Velocity (fps)"=0.0, "Accel (fps^2)"=0.0, "Jerk (fps^3)"=0.0, "StoopidFast (fps)"=0.0}, "Conditions"={"vInitial (fps)"=0.0, "vFinal (fps)"=0.0}, "Overrides"=[], "Angular Limits"={"Velocity (deg/s)"=0.0, "Accel (deg/s^2)"=0.0, "Jerk (deg/s^3)"=0.0}} ("output cluster"), 11:w356) -> (2:w370:T23, 3:w369:refnum<file>)  [unwired: 4 in, 2 out]
      n120 = Unbundle(w370) -> ("Sample Period (s)"=w333:dbl, "Limits"=w354:T22, "Conditions"=w364:T27, "Overrides"=w343:T5, "Angular Limits"=w342:T6)
      n121 = Read from Binary File(5:w368, 11:w369) -> (2:w367:cluster{"x":dbl, "y":dbl, "th":dbl}[], 3:w359:refnum<file>)  [unwired: 4 in, 2 out]
      n122 = Read from Binary File(5:w365, 11:w359) -> (2:w345:cluster{"Time (s)":dbl, "Distance (ft)":dbl}, 3:w348:refnum<file>)  [unwired: 4 in, 2 out]
      n123 = Unbundle(w354) -> ("Velocity (fps)"=w352:dbl, "Accel (fps^2)"=w351:dbl, "Jerk (fps^3)"=w350:dbl, "StoopidFast (fps)"=w349:dbl)
      n124 = Bundle("Velocity (fps)"=w352, "Accel (fps^2)"=w351, "Jerk (fps^3)"=w350, "StoopidFast (fps)"=w349) -> (w353:T33)  [unwired: 1 in]
      n125 = Read from Binary File(5:FALSE, 11:w348) -> (2:w346:bool, 3:w341:refnum<file>)  [unwired: 4 in, 2 out]
      n126 = Read from Binary File(5:cluster{"Drive Type":T3, "Path Type":T4} {"Drive Type"=enum."Nonholonomic", "Path Type"=enum."Clothoid"} ("Trajectory Meta"), 11:w341) -> (2:w338:cluster{"Drive Type":T3, "Path Type":T4}, 3:w339:refnum<file>)  [unwired: 4 in, 2 out]
      n127 = call "Convert Command Data 5.0.vi"("Pre 5.0 Command Data"=w335) -> ("5.0 Command Data"=w334:T8)  [unwired: 10 in]
    }
    frame "4.0" {
      # "Adding the zeroV overriede"
      n128 = Read from Binary File(5:T11 {"Robot Backwards"=FALSE, "Reverse Path"=FALSE} ("Cluster"), 11:w399) -> (2:w393:T11, 3:w396:refnum<file>)  [unwired: 4 in, 2 out]
      n129 = Read from Binary File(5:w375, 11:w396) -> (2:w401:T1, 3:w395:refnum<file>)  [unwired: 4 in, 2 out]
      n130 = Read from Binary File(5:cluster{"Time (s)":dbl, T9, bool}[] [] ("Commands in"), 11:w395) -> (0:w400:errorcluster, 2:w373:cluster{"Time (s)":dbl, T9, bool}[], 3:w394:refnum<file>)  [unwired: 4 in, 1 out]
      n131 = Read from Binary File(5:T23 {"Sample Period (s)"=0.0, "Limits"={"Velocity (fps)"=0.0, "Accel (fps^2)"=0.0, "Jerk (fps^3)"=0.0, "StoopidFast (fps)"=0.0}, "Conditions"={"vInitial (fps)"=0.0, "vFinal (fps)"=0.0}, "Overrides"=[], "Angular Limits"={"Velocity (deg/s)"=0.0, "Accel (deg/s^2)"=0.0, "Jerk (deg/s^3)"=0.0}} ("output cluster"), 11:w394) -> (2:w407:T23, 3:w406:refnum<file>)  [unwired: 4 in, 2 out]
      n132 = Unbundle(w407) -> ("Sample Period (s)"=w372:dbl, "Limits"=w392:T22, "Conditions"=w402:T27, "Overrides"=w381:T5, "Angular Limits"=w380:T6)
      n133 = Read from Binary File(5:w405, 11:w406) -> (2:w404:cluster{"x":dbl, "y":dbl, "th":dbl}[], 3:w397:refnum<file>)  [unwired: 4 in, 2 out]
      n134 = Read from Binary File(5:w403, 11:w397) -> (2:w383:cluster{"Time (s)":dbl, "Distance (ft)":dbl}, 3:w386:refnum<file>)  [unwired: 4 in, 2 out]
      n135 = Unbundle(w392) -> ("Velocity (fps)"=w390:dbl, "Accel (fps^2)"=w389:dbl, "Jerk (fps^3)"=w388:dbl, "StoopidFast (fps)"=w387:dbl)
      n136 = Bundle("Velocity (fps)"=w390, "Accel (fps^2)"=w389, "Jerk (fps^3)"=w388, "StoopidFast (fps)"=w387) -> (w391:T33)  [unwired: 1 in]
      n137 = Read from Binary File(5:FALSE, 11:w386) -> (2:w384:bool, 3:w379:refnum<file>)  [unwired: 4 in, 2 out]
      n138 = Read from Binary File(5:cluster{"Drive Type":T3, "Path Type":T4} {"Drive Type"=enum."Nonholonomic", "Path Type"=enum."Clothoid"} ("Trajectory Meta"), 11:w379) -> (2:w376:cluster{"Drive Type":T3, "Path Type":T4}, 3:w377:refnum<file>)  [unwired: 4 in, 2 out]
      n139 = call "Convert Command Data 5.0.vi"("Pre 5.0 Command Data"=w373) -> ("5.0 Command Data"=w371:T8)  [unwired: 10 in]
    }
    frame "4.2" {
      # "Adding the zeroV overriede"
      n140 = Read from Binary File(5:T11 {"Robot Backwards"=FALSE, "Reverse Path"=FALSE} ("Cluster"), 11:w439) -> (2:w433:T11, 3:w436:refnum<file>)  [unwired: 4 in, 2 out]
      n141 = Read from Binary File(5:w416, 11:w436) -> (2:w441:T1, 3:w435:refnum<file>)  [unwired: 4 in, 2 out]
      n142 = Read from Binary File(5:cluster{"Time (s)":dbl, T9, bool}[] [] ("Commands in"), 11:w435) -> (0:w440:errorcluster, 2:w410:cluster{"Time (s)":dbl, T9, bool}[], 3:w434:refnum<file>)  [unwired: 4 in, 1 out]
      n143 = Read from Binary File(5:T23 {"Sample Period (s)"=0.0, "Limits"={"Velocity (fps)"=0.0, "Accel (fps^2)"=0.0, "Jerk (fps^3)"=0.0, "StoopidFast (fps)"=0.0}, "Conditions"={"vInitial (fps)"=0.0, "vFinal (fps)"=0.0}, "Overrides"=[], "Angular Limits"={"Velocity (deg/s)"=0.0, "Accel (deg/s^2)"=0.0, "Jerk (deg/s^3)"=0.0}} ("output cluster"), 11:w434) -> (2:w447:T23, 3:w446:refnum<file>)  [unwired: 4 in, 2 out]
      n144 = Read from Binary File(5:w445, 11:w446) -> (2:w444:cluster{"x":dbl, "y":dbl, "th":dbl}[], 3:w437:refnum<file>)  [unwired: 4 in, 2 out]
      n145 = Unbundle(w447) -> ("Sample Period (s)"=w408:dbl, "Limits"=w432:T22, "Conditions"=w442:T27, "Overrides"=w421:T5, "Angular Limits"=w420:T6)
      n146 = Read from Binary File(5:w443, 11:w437) -> (2:w423:cluster{"Time (s)":dbl, "Distance (ft)":dbl}, 3:w426:refnum<file>)  [unwired: 4 in, 2 out]
      n147 = Unbundle(w432) -> ("Velocity (fps)"=w430:dbl, "Accel (fps^2)"=w429:dbl, "Jerk (fps^3)"=w428:dbl, "StoopidFast (fps)"=w427:dbl)
      n148 = Read from Binary File(5:FALSE, 11:w426) -> (2:w424:bool, 3:w419:refnum<file>)  [unwired: 4 in, 2 out]
      n149 = Bundle("Velocity (fps)"=w430, "Accel (fps^2)"=w429, "Jerk (fps^3)"=w428, "StoopidFast (fps)"=w427) -> (w431:T33)  [unwired: 1 in]
      n150 = Read from Binary File(5:cluster{"Drive Type":T3, "Path Type":T4} {"Drive Type"=enum."Nonholonomic", "Path Type"=enum."Clothoid"} ("Trajectory Meta"), 11:w419) -> (2:w417:cluster{"Drive Type":T3, "Path Type":T4}, 3:w415:refnum<file>)  [unwired: 4 in, 2 out]
      n151 = Read from Binary File(5:FALSE, 11:w415) -> (2:w412:bool, 3:w414:refnum<file>)  [unwired: 4 in, 2 out]
      n152 = call "Convert Command Data 5.0.vi"("Pre 5.0 Command Data"=w410) -> ("5.0 Command Data"=w409:T8)  [unwired: 10 in]
    }
    frame "4.3" {
      # "Adding the zeroV overriede"
      n153 = Read from Binary File(5:T11 {"Robot Backwards"=FALSE, "Reverse Path"=FALSE} ("Cluster"), 11:w482) -> (2:w476:T11, 3:w479:refnum<file>)  [unwired: 4 in, 2 out]
      n154 = Read from Binary File(5:w459, 11:w479) -> (2:w484:T1, 3:w478:refnum<file>)  [unwired: 4 in, 2 out]
      n155 = Read from Binary File(5:cluster{"Time (s)":dbl, T9, bool}[] [] ("Commands in"), 11:w478) -> (0:w483:errorcluster, 2:w450:cluster{"Time (s)":dbl, T9, bool}[], 3:w477:refnum<file>)  [unwired: 4 in, 1 out]
      n156 = Read from Binary File(5:T23 {"Sample Period (s)"=0.0, "Limits"={"Velocity (fps)"=0.0, "Accel (fps^2)"=0.0, "Jerk (fps^3)"=0.0, "StoopidFast (fps)"=0.0}, "Conditions"={"vInitial (fps)"=0.0, "vFinal (fps)"=0.0}, "Overrides"=[], "Angular Limits"={"Velocity (deg/s)"=0.0, "Accel (deg/s^2)"=0.0, "Jerk (deg/s^3)"=0.0}} ("output cluster"), 11:w477) -> (2:w490:T23, 3:w489:refnum<file>)  [unwired: 4 in, 2 out]
      n157 = Read from Binary File(5:w488, 11:w489) -> (2:w487:cluster{"x":dbl, "y":dbl, "th":dbl}[], 3:w480:refnum<file>)  [unwired: 4 in, 2 out]
      n158 = Unbundle(w490) -> ("Sample Period (s)"=w448:dbl, "Limits"=w475:T22, "Conditions"=w485:T27, "Overrides"=w464:T5, "Angular Limits"=w463:T6)
      n159 = Read from Binary File(5:w486, 11:w480) -> (2:w466:cluster{"Time (s)":dbl, "Distance (ft)":dbl}, 3:w469:refnum<file>)  [unwired: 4 in, 2 out]
      n160 = Unbundle(w475) -> ("Velocity (fps)"=w473:dbl, "Accel (fps^2)"=w472:dbl, "Jerk (fps^3)"=w471:dbl, "StoopidFast (fps)"=w470:dbl)
      n161 = Read from Binary File(5:FALSE, 11:w469) -> (2:w467:bool, 3:w462:refnum<file>)  [unwired: 4 in, 2 out]
      n162 = Bundle("Velocity (fps)"=w473, "Accel (fps^2)"=w472, "Jerk (fps^3)"=w471, "StoopidFast (fps)"=w470) -> (w474:T33)  [unwired: 1 in]
      n163 = Read from Binary File(5:cluster{"Drive Type":T3, "Path Type":T4} {"Drive Type"=enum."Nonholonomic", "Path Type"=enum."Clothoid"} ("Trajectory Meta"), 11:w462) -> (2:w460:cluster{"Drive Type":T3, "Path Type":T4}, 3:w458:refnum<file>)  [unwired: 4 in, 2 out]
      n164 = Read from Binary File(5:FALSE, 11:w458) -> (2:w456:bool, 3:w455:refnum<file>)  [unwired: 4 in, 2 out]
      n165 = Read from Binary File(5:0.0, 11:w455) -> (2:w452:dbl, 3:w454:refnum<file>)  [unwired: 4 in, 2 out]
      n166 = call "Convert Command Data 5.0.vi"("Pre 5.0 Command Data"=w450) -> ("5.0 Command Data"=w449:T8)  [unwired: 10 in]
    }
    frame "4.4" {
      w498 = FALSE
      # "Adding the zeroV overriede"
      n167 = Read from Binary File(5:T11 {"Robot Backwards"=FALSE, "Reverse Path"=FALSE} ("Cluster"), 11:w530) -> (2:w524:T11, 3:w527:refnum<file>)  [unwired: 4 in, 2 out]
      n168 = Read from Binary File(5:w507, 11:w527) -> (2:w532:T1, 3:w526:refnum<file>)  [unwired: 4 in, 2 out]
      n169 = Read from Binary File(5:cluster{"Time (s)":dbl, T9, bool}[] [] ("Commands in"), 11:w526) -> (0:w531:errorcluster, 2:w492:cluster{"Time (s)":dbl, T9, bool}[], 3:w525:refnum<file>)  [unwired: 4 in, 1 out]
      n170 = Read from Binary File(5:T23 {"Sample Period (s)"=0.0, "Limits"={"Velocity (fps)"=0.0, "Accel (fps^2)"=0.0, "Jerk (fps^3)"=0.0, "StoopidFast (fps)"=0.0}, "Conditions"={"vInitial (fps)"=0.0, "vFinal (fps)"=0.0}, "Overrides"=[], "Angular Limits"={"Velocity (deg/s)"=0.0, "Accel (deg/s^2)"=0.0, "Jerk (deg/s^3)"=0.0}} ("output cluster"), 11:w525) -> (2:w538:T23, 3:w537:refnum<file>)  [unwired: 4 in, 2 out]
      n171 = Read from Binary File(5:w536, 11:w537) -> (2:w535:cluster{"x":dbl, "y":dbl, "th":dbl}[], 3:w528:refnum<file>)  [unwired: 4 in, 2 out]
      n172 = Unbundle(w538) -> ("Sample Period (s)"=w491:dbl, "Limits"=w523:T22, "Conditions"=w533:T27, "Overrides"=w512:T5, "Angular Limits"=w511:T6)
      n173 = Read from Binary File(5:w534, 11:w528) -> (2:w514:cluster{"Time (s)":dbl, "Distance (ft)":dbl}, 3:w517:refnum<file>)  [unwired: 4 in, 2 out]
      n174 = Unbundle(w523) -> ("Velocity (fps)"=w521:dbl, "Accel (fps^2)"=w520:dbl, "Jerk (fps^3)"=w519:dbl, "StoopidFast (fps)"=w518:dbl)
      n175 = Read from Binary File(5:FALSE, 11:w517) -> (2:w515:bool, 3:w510:refnum<file>)  [unwired: 4 in, 2 out]
      n176 = Bundle("Velocity (fps)"=w521, "Accel (fps^2)"=w520, "Jerk (fps^3)"=w519, "StoopidFast (fps)"=w518) -> (w522:T33)  [unwired: 1 in]
      n177 = Read from Binary File(5:cluster{"Drive Type":T3, "Path Type":T4} {"Drive Type"=enum."Nonholonomic", "Path Type"=enum."Clothoid"} ("Trajectory Meta"), 11:w510) -> (2:w508:cluster{"Drive Type":T3, "Path Type":T4}, 3:w506:refnum<file>)  [unwired: 4 in, 2 out]
      n178 = Read from Binary File(5:FALSE, 11:w506) -> (2:w504:bool, 3:w503:refnum<file>)  [unwired: 4 in, 2 out]
      n179 = Read from Binary File(5:0.0, 11:w503) -> (2:w501:dbl, 3:w500:refnum<file>)  [unwired: 4 in, 2 out]
      n180 = Read from Binary File(5:w498, 11:w500) -> (2:w497:bool, 3:w499:refnum<file>)  [unwired: 4 in, 2 out]
      n181 = Read from Binary File(5:w498, 11:w499) -> (2:w496:bool, 3:w495:refnum<file>)  [unwired: 4 in, 2 out]
      n182 = call "Convert Command Data 5.0.vi"("Pre 5.0 Command Data"=w492) -> ("5.0 Command Data"=w493:T8)  [unwired: 10 in]
    }
    frame "5.0" {
      # "Adding the zeroV overriede"
      n183 = Read from Binary File(5:T11 {"Robot Backwards"=FALSE, "Reverse Path"=FALSE} ("Cluster"), 11:w571) -> (2:w565:T11, 3:w568:refnum<file>)  [unwired: 4 in, 2 out]
      n184 = Read from Binary File(5:w547, 11:w568) -> (2:w574:T1, 3:w567:refnum<file>)  [unwired: 4 in, 2 out]
      n185 = Read from Binary File(5:T24 data[4990B] ("Commands"), 11:w567) -> (0:w572:errorcluster, 2:w573:T24, 3:w566:refnum<file>)  [unwired: 4 in, 1 out]
      n186 = Read from Binary File(5:T23 {"Sample Period (s)"=0.0, "Limits"={"Velocity (fps)"=0.0, "Accel (fps^2)"=0.0, "Jerk (fps^3)"=0.0, "StoopidFast (fps)"=0.0}, "Conditions"={"vInitial (fps)"=0.0, "vFinal (fps)"=0.0}, "Overrides"=[], "Angular Limits"={"Velocity (deg/s)"=0.0, "Accel (deg/s^2)"=0.0, "Jerk (deg/s^3)"=0.0}} ("output cluster"), 11:w566) -> (2:w580:T23, 3:w579:refnum<file>)  [unwired: 4 in, 2 out]
      n187 = Read from Binary File(5:w578, 11:w579) -> (2:w577:cluster{"x":dbl, "y":dbl, "th":dbl}[], 3:w569:refnum<file>)  [unwired: 4 in, 2 out]
      n188 = Unbundle(w580) -> ("Sample Period (s)"=w558:dbl, "Limits"=w564:T22, "Conditions"=w575:T27, "Overrides"=w552:T5, "Angular Limits"=w551:T6)
      n189 = Read from Binary File(5:w576, 11:w569) -> (2:w554:cluster{"Time (s)":dbl, "Distance (ft)":dbl}, 3:w557:refnum<file>)  [unwired: 4 in, 2 out]
      n190 = Unbundle(w564) -> ("Velocity (fps)"=w562:dbl, "Accel (fps^2)"=w561:dbl, "Jerk (fps^3)"=w560:dbl, "StoopidFast (fps)"=w559:dbl)
      n191 = Read from Binary File(5:FALSE, 11:w557) -> (2:w555:bool, 3:w550:refnum<file>)  [unwired: 4 in, 2 out]
      n192 = Bundle("Velocity (fps)"=w562, "Accel (fps^2)"=w561, "Jerk (fps^3)"=w560, "StoopidFast (fps)"=w559) -> (w563:T33)  [unwired: 1 in]
      n193 = Read from Binary File(5:cluster{"Drive Type":T3, "Path Type":T4} {"Drive Type"=enum."Nonholonomic", "Path Type"=enum."Clothoid"} ("Trajectory Meta"), 11:w550) -> (2:w548:cluster{"Drive Type":T3, "Path Type":T4}, 3:w540:refnum<file>)  [unwired: 4 in, 2 out]
      n194 = Read from Binary File(5:0.0, 11:w540) -> (2:w545:dbl, 3:w544:refnum<file>)  [unwired: 4 in, 2 out]
      n195 = Read from Binary File(5:FALSE, 11:w544) -> (2:w542:bool, 3:w541:refnum<file>)  [unwired: 4 in, 2 out]
    }
  }
  "Zero V" <- w21
  "Reversals" <- w20
  "Commands out" <- w18
  "Points out" <- w17
  "Overall" <- w9
  "Trajectory Meta" <- w6
  "Trajectory Data" <- w3
  "Current Limit" <- w2
  "Zero Translational Velocity" <- w1
  n196 = Bundle("Sample Period (s)"=w23, w24, "Conditions"=w25, "Overrides"=w26, "Angular Limits"=w7) -> (→"Fields":T7)  [unwired: 1 in]
  n197 = Close File(refnum=w14) -> ()  [unwired: 1 in, 2 out]
